vi "P4CMD Dialog_CheckProjData.vi"(7 "P4Proj UIDialog FP Refs":T1, 8 "error in (no error)":errorcluster, 10 "use defaults? (F)":bool) -> (0 "error out":errorcluster)   [LabVIEW 2020, in "NI_SCC_P4CMD.lvlib"]
uses:
  <vilib>/SourceControl/Providers/P4CMD/NI_SCC_P4CMD.lvlib
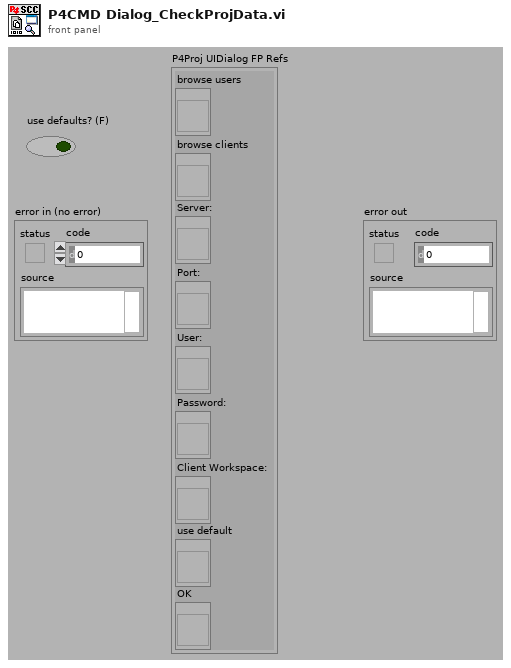
[diagram p1: front panel]
types:
  T1 = cluster{"browse users":refnum<vi>, "browse clients":refnum<vi>, "Server:":refnum<vi>, "Port:":refnum<vi>, "User:":refnum<vi>, "Password:":refnum<vi>, "Client Workspace:":refnum<vi>, "use default":refnum<vi>, "OK":refnum<vi>}
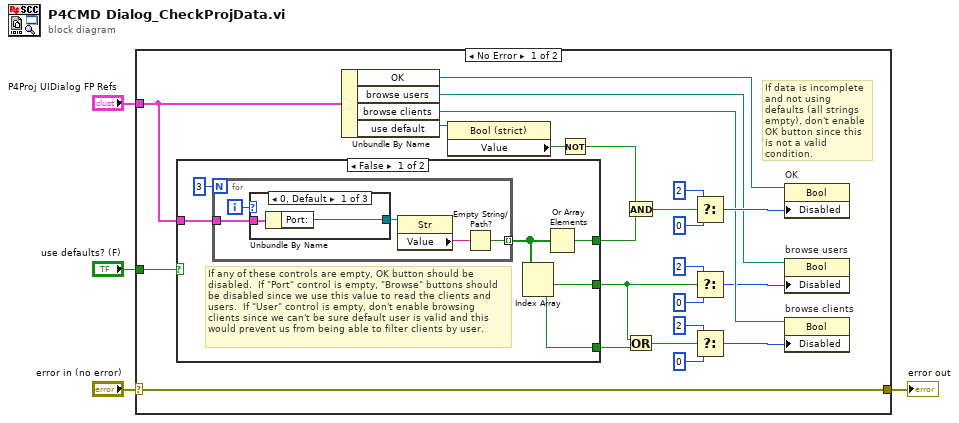
[diagram p0: block diagram]
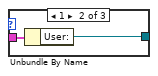
[diagram p2: hidden frame]
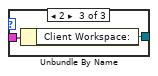
[diagram p3: hidden frame]
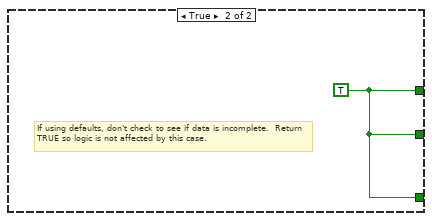
[diagram p4: hidden frame]
diagram:
  n1 = case shown="No Error" "error in (no error)" {
    selector: "error in (no error)" -> [w12 w46]
    tunnel: "P4Proj UIDialog FP Refs" -> [w21 _]
    tunnel: [w12 w46] -> w2
    tunnel: "use defaults? (F)" -> [w5 _]
    frame No Error {
      # "If data is incomplete and not using defaults (all strings empty), don't enable OK button since this is not a valid condition."
      n2 = case shown="False" w5 {
        tunnel: [w31 w45] -> w27
        tunnel: w21 -> [w30 _]
        tunnel: [w29 w45] -> w7
        tunnel: [w28 w45] -> w6
        frame False {
          # "If any of these controls are empty, OK button should be disabled.  If \"Port\" control is empty, \"Browse\" buttons should be disabled since we use this value to read the clients and users.  If \"User\" control is empty, don't enable browsing clients since we can't be sure default user is valid and this would prevent us from being able to filter clients by user."
          n3 = for {
            N: 3 -> [_]
            tunnel: w30 -> [w38]
            tunnel: [w36] -> w32 mode=indexing
            i -> [w37]
            n4 = case shown="0, Default" w37 {
              tunnel: w38 -> [w40 w42 w44]
              tunnel: [w39 w41 w43] -> w35
              frame 0, Default {
                n5 = Unbundle By Name(w40) -> ("Port:"=w39:refnum<vi>)
              }
              frame 1 {
                n6 = Unbundle By Name(w42) -> ("User:"=w41:refnum<vi>)
              }
              frame 2 {
                n7 = Unbundle By Name(w44) -> ("Client Workspace:"=w43:refnum<vi>)
              }
            }
            n8 = property class="Str"(reference=w35) -> ("Value"=w34:string)  [unwired: 1 in, 2 out]
            n9 = Empty String/Path?(string/path=w34) -> (empty?=w36:bool)
          }
          n10 = Index Array(array=w32) -> (element #1=w29:bool, element #2=w28:bool)  [unwired: 2 in]
          n11 = Or Array Elements(Boolean array=w32) -> (logical OR=w31:bool)
        }
        frame True {
          w45 = TRUE
          # "If using defaults, don't check to see if data is incomplete.  Return TRUE so logic is not affected by this case."
        }
      }
      n12 = Unbundle By Name(w21) -> ("OK"=w20:refnum<vi>, "browse users"=w18:refnum<vi>, "browse clients"=w17:refnum<vi>, "use default"=w14:refnum<vi>)
      n13 = property class="Bool (strict)"(reference=w14) -> ("Value"=w13:bool)  [unwired: 1 in, 2 out]
      n14 = Not(x=w13) -> (.not. x?=w15:bool)
      n15 = And(x=w15, y=w27) -> (x .and. y?=w22:bool)
      n16 = Or(x=w7, y=w6) -> (x .or. y?=w8:bool)
      n17 = Select(t=u8 2 ("Disabled"), s=w22, f=u8 0) -> (s? t:f=w19:u8)
      n18 = Select(t=u8 2 ("Disabled"), s=w7, f=u8 0) -> (s? t:f=w16:u8)
      n19 = Select(t=u8 2 ("Disabled"), s=w8, f=u8 0) -> (s? t:f=w9:u8)
      n20 = property on="OK" class="Bool"(reference=w20, "Disabled"=w19) -> ()  [unwired: 1 in, 2 out]
      n21 = property on="browse users" class="Bool"(reference=w18, "Disabled"=w16) -> ()  [unwired: 1 in, 2 out]
      n22 = property on="browse clients" class="Bool"(reference=w17, "Disabled"=w9) -> ()  [unwired: 1 in, 2 out]
    }
    frame Error {
    }
  }
  "error out" <- w2
